vi "HCC Filter NonUsed Agilent Channels.vi"(8 "Error In":errorcluster, 9 "Disable Channel = True":bool[](array[boolean]), 10 "Input Current":dbl[](array[numeric]) format="%.2f", 11 "Voltage Indexes":i32[](array[numeric])) -> (0 "Error Out":errorcluster, 2 "Output Voltage":dbl[](array[numeric]), 3 "Output Current":dbl[](array[numeric]))   [LabVIEW 2016]
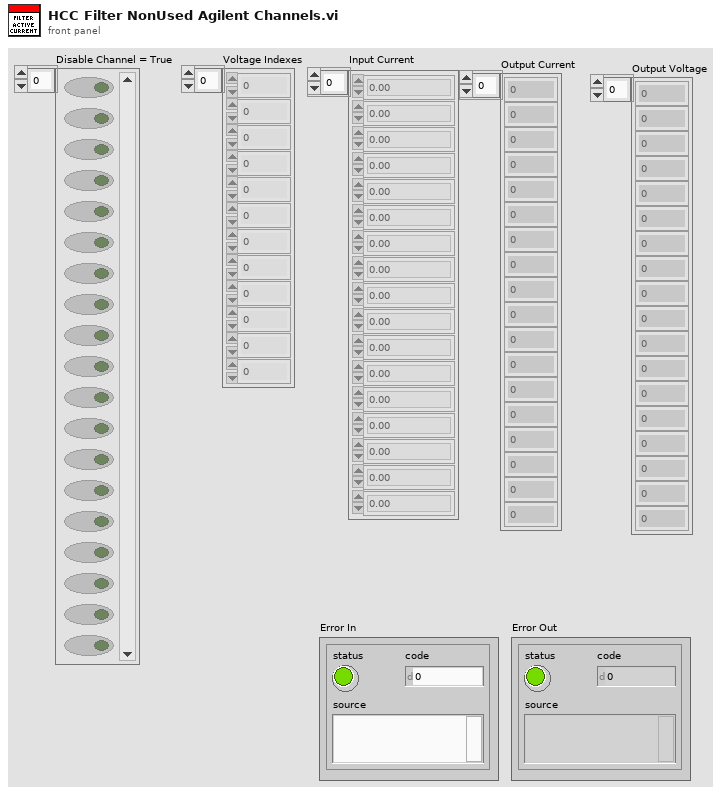
[diagram p1: front panel]
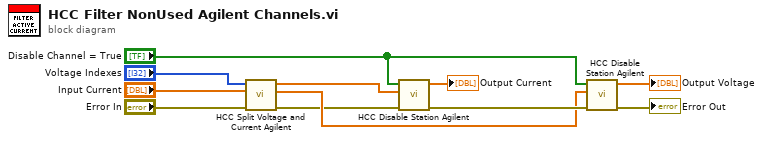
[diagram p0: block diagram]
diagram:
  n1 = call "HCC Split Voltage and Current Agilent.vi"("Error In"="Error In", "Input Agilent Array"="Input Current", "Voltage Indexes"="Voltage Indexes") -> ("Error Out"=w2:errorcluster, "Voltage Array"=w5:dbl[], "Current Array"=w6:dbl[])  [unwired: 6 in]
  n2 = call "HCC Disable Station Agilent.vi"("Error In"=w2, "Raw Input Array"=w6, "Disable Channel = True"="Disable Channel = True") -> ("Error Out"=w8:errorcluster, "Corrected Array"=→"Output Current":dbl[])  [unwired: 7 in]
  n3 = call "HCC Disable Station Agilent.vi"("Error In"=w8, "Raw Input Array"=w5, "Disable Channel = True"="Disable Channel = True") -> ("Error Out"=→"Error Out":errorcluster, "Corrected Array"=→"Output Voltage":dbl[])  [unwired: 7 in]
